vi "PathMakerPNGSaver_.vi"(4 "Height":T1, 6 "Reflectivity":T1, 8 "patterns":i32, 9 "frame number":i32, 11 "path":path=path "C:/Users/optics/Documents/Matt/Time Of Flight/Data/20150722") -> (2 "Height path":path, 3 "Reflectivity path":path)   [LabVIEW 2020]
uses:
  <vilib>/picture/picture.llb/imagedata.ctl
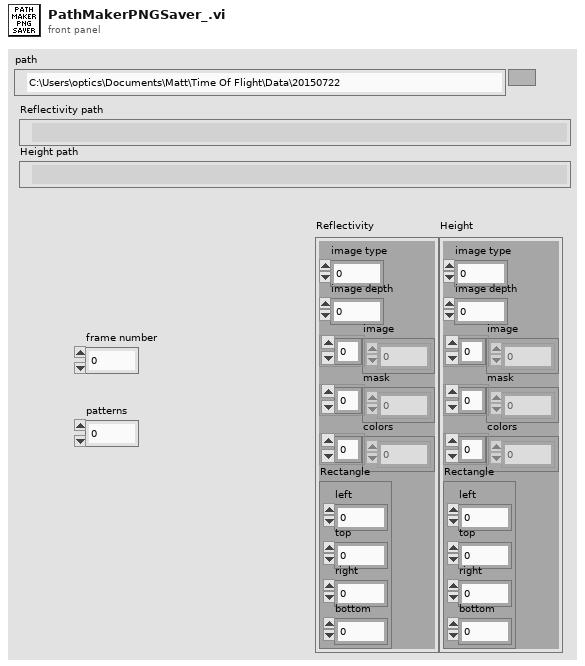
[diagram p1: front panel]
types:
  T1 = typedef "imagedata.ctl" = cluster{"image type":i32, "image depth":i32, "image":u8[], "mask":u8[], "colors":u32[], "Rectangle":cluster{"left":i16, "top":i16, "right":i16, "bottom":i16}}
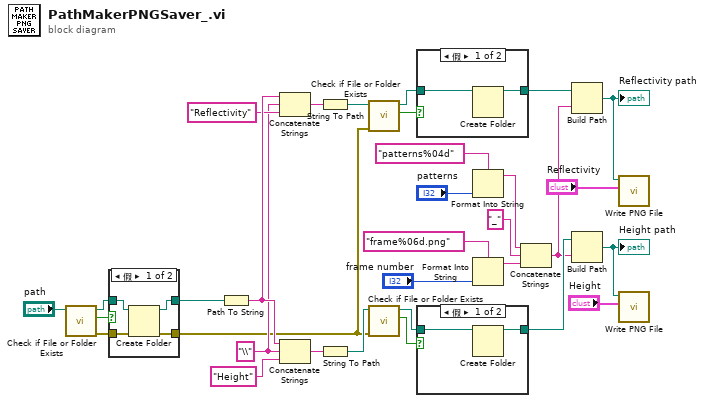
[diagram p0: block diagram]
diagram:
  w27 = "\\" ("string")
  n1 = call <vilib>:"Check if File or Folder Exists.vi"("path"="path") -> ("error out"=w23:errorcluster, "file or folder exists?"=w25:bool, "dup path"=w24:path)  [unwired: 8 in]
  n2 = case shown="假" w25 {
    tunnel: [w36 w38] -> w22
    tunnel: w24 -> [w35 w38]
    tunnel: w23 -> [w34 w37]
    tunnel: [w33 w37] -> w19
    frame False {
      n3 = Create Folder(path (use dialog)=w35, error in=w34) -> (created path=w36:path, error out=w33:errorcluster)  [unwired: 1 in, 1 out]
    }
    frame True {
    }
  }
  n4 = Path To String(path=w22) -> (string=w32:string)
  n5 = Concatenate Strings(w32, w27, "Reflectivity" ("string")) -> (w28:string)
  n6 = Concatenate Strings(w32, w27, "Height" ("string")) -> (w31:string)
  n7 = String To Path(string=w28) -> (path=w20:path)
  n8 = String To Path(string=w31) -> (path=w21:path)
  n9 = call <vilib>:"Check if File or Folder Exists.vi"("error in (no error)"=w19, "path"=w20) -> ("file or folder exists?"=w18:bool, "dup path"=w16:path)  [unwired: 7 in, 1 out]
  n10 = call <vilib>:"Check if File or Folder Exists.vi"("error in (no error)"=w19, "path"=w21) -> ("file or folder exists?"=w17:bool, "dup path"=w15:path)  [unwired: 7 in, 1 out]
  n11 = case shown="假" w18 {
    tunnel: w16 -> [w40 w41]
    tunnel: [w39 w41] -> w6
    frame False {
      n12 = Create Folder(path (use dialog)=w40) -> (created path=w39:path)  [unwired: 2 in, 2 out]
    }
    frame True {
    }
  }
  n13 = case shown="假" w17 {
    tunnel: w15 -> [w43 w44]
    tunnel: [w42 w44] -> w7
    frame False {
      n14 = Create Folder(path (use dialog)=w43) -> (created path=w42:path)  [unwired: 2 in, 2 out]
    }
    frame True {
    }
  }
  n15 = Format Into String(format string="patterns%04d", "patterns") -> (resulting string=w9:string)  [unwired: 2 in, 1 out]
  n16 = Format Into String(format string="frame%06d.png", "frame number") -> (resulting string=w8:string)  [unwired: 2 in, 1 out]
  n17 = Concatenate Strings(w9, "_" ("string"), w8) -> (w5:string)
  n18 = Build Path(base path=w6, name or relative path=w5) -> (appended path=w2:path)
  "Reflectivity path" <- w2
  n19 = Build Path(base path=w7, name or relative path=w5) -> (appended path=w1:path)
  "Height path" <- w1
  n20 = call <vilib>:"Write PNG File.vi"("image data"="Reflectivity", "path to PNG file"=w2) -> ()  [unwired: 8 in, 2 out]
  n21 = call <vilib>:"Write PNG File.vi"("image data"="Height", "path to PNG file"=w1) -> ()  [unwired: 8 in, 2 out]
